vi "LC GetConrolName.vi"(8 "error in (no error)":errorcluster caption="Error In", 10 "VI Path":path, 11 "Treeref":refnum<vi>) -> (0 "error out":errorcluster caption="Error Out", 2 "Control Path Out":string[](array[string]), 3 "Ctl Ref Out":refnum<vi>[](array[refnum]))   [LabVIEW 2020]
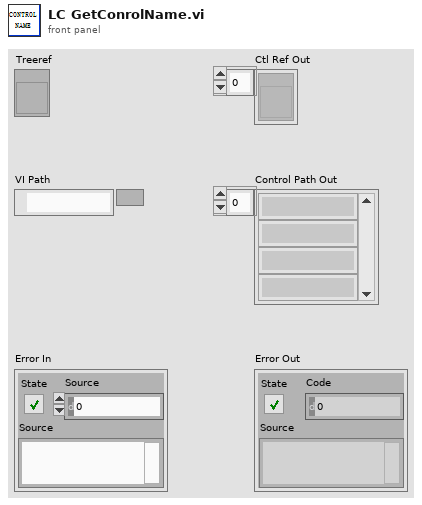
[diagram p1: front panel]
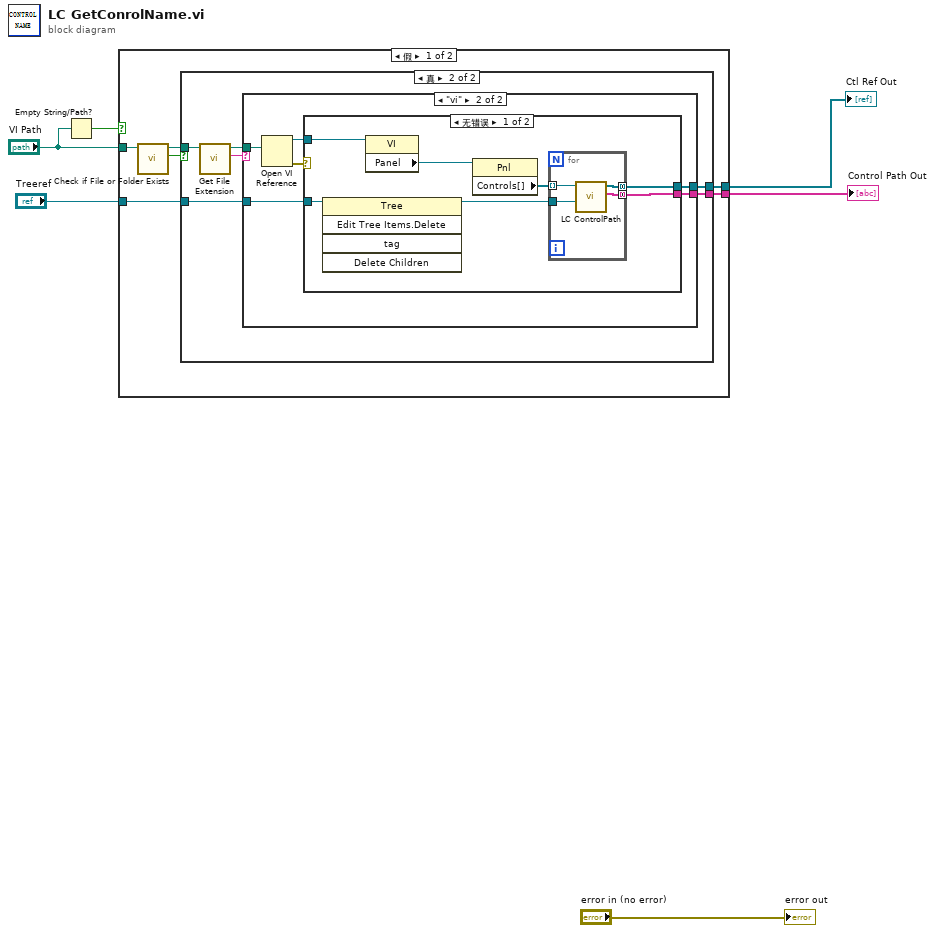
[diagram p0: block diagram]
diagram:
  n1 = Empty String/Path?(string/path="VI Path") -> (empty?=w4:bool)
  n2 = case shown="假" w4 {
    tunnel: "VI Path" -> [w12 _]
    tunnel: "Treeref" -> [w9 _]
    tunnel: [w8 _] -> w1
    tunnel: [w7 _] -> w2
    frame False {
      n3 = call <vilib>:"Check if File or Folder Exists.vi"("path"=w12) -> ("file or folder exists?"=w10:bool, "dup path"=w11:path)  [unwired: 8 in, 1 out]
      n4 = case shown="真" w10 {
        tunnel: w11 -> [_ w17]
        tunnel: w9 -> [_ w18]
        tunnel: [_ w14] -> w8
        tunnel: [_ w13] -> w7
        frame False {
        }
        frame True {
          n5 = call <vilib>:"Get File Extension.vi"("file"=w17) -> ("lowercase file extension"=w15:string, "dup file"=w16:path)  [unwired: 6 in, 3 out]
          n6 = case shown="\"vi\"" w15 {
            tunnel: w18 -> [_ w22]
            tunnel: w16 -> [_ w21]
            tunnel: [_ w20] -> w14
            tunnel: [_ w19] -> w13
            frame "假", Default {
            }
            frame "vi" {
              n7 = Open VI Reference(vi path=w21) -> (vi reference=w24:refnum<vi>, error out=w23:errorcluster)  [unwired: 5 in]
              n8 = case shown="无错误" w23 {
                tunnel: w24 -> [w29 _]
                tunnel: w22 -> [w27 _]
                tunnel: [w26 _] -> w20
                tunnel: [w25 _] -> w19
                frame No Error {
                  n9 = invoke class="Tree" method="Edit Tree Items.Delete"(reference=w27) -> (reference out=w28:refnum<vi>)  [unwired: 4 in, 4 out]
                  n10 = property class="VI"(reference=w29) -> ("Panel"=w30:refnum<vi>)  [unwired: 1 in, 2 out]
                  n11 = property class="Pnl"(reference=w30) -> ("Controls[]"=w31:refnum<vi>[])  [unwired: 1 in, 2 out]
                  n12 = for {
                    tunnel: w31 -> [w35] mode=indexing
                    tunnel: w28 -> [w34]
                    tunnel: [w33] -> w26 mode=concatenating
                    tunnel: [w32] -> w25 mode=concatenating
                    n13 = call "LC ControlPath.vi"("Treeref"=w34, "Ctl Ref In"=w35) -> ("Control Path Out"=w33:string[], "Ctl Ref Out"=w32:refnum<vi>[])  [unwired: 7 in, 1 out]
                  }
                }
                frame Error {
                }
              }
            }
          }
        }
      }
    }
    frame True {
    }
  }
  "Ctl Ref Out" <- w2
  "Control Path Out" <- w1
  "error out" <- "error in (no error)"
